vi "EEG Preprocessing.vi"() -> ()   [LabVIEW 2016]
uses:
  3. Features Extraction/_Feature Extraction Utility/_vlib/EF_FrequencyFilter.ctl
  3. Features Extraction/_Feature Extraction Utility/_vlib/EF_SpatialFilter.ctl
  _XML_EEG_File_Parser/_vlib/XML_EEG_File.lvclass
  <vilib>/xml/Load XML File.vi
  <vilib>/xml/NI_XML.lvlib
  3. Features Extraction/_Feature Extraction Utility/Feature Extraction.lvlib
panel:
  in  "Apply Settings":bool
  in  "Tab Control 2":T1(tab)=enum."Частотная фильтрация"
  in  "EOG channels":i32[](array[numeric])=[22, 23, 24] caption="Каналы с электроокулограммой (ЭОГ)" min=0 max=256 step=1
  in  "CSP params":path caption="Путь к файлу с параметрами CSP-фильтра"
  in  "SpatialFilter":T2=enum."Common Average Reference" caption="Метод пространственной фильтрации"
  in  "low cutoff freq":dbl=0.5 caption="Нижняя граница полосы пропускания, Гц"
  in  "high cutoff freq":dbl=50.0 caption="Верхняя граница полосы пропускания, Гц"
  in  "FrequencyFilter":T3 caption="Метод частотной фильтрации"
  in  "ReInit?":bool
  in  "Exit Button":bool
  in  "Tab Control":enum32{"Сигнал ЭЭГ", "Один канал"}(tab)
  out "Class Label":string caption="Метка класса"
  out "Dataset Number":i32 caption="Номер пробы"
  out "Raw EEG":dbl[][](graph) caption="Сигнал ЭЭГ (ориг.)"
  out "Preprocessed EEG":dbl[][](graph) caption="Сигнал ЭЭГ после предобработки"
  in  "Next Dataset":bool
  in  "Previous Dataset":bool
  out "Channel Name":string caption="Название канала"
  in  "Channel Number":i32 caption="Номер канала" min=0 max=24 step=1
  out "Wavelet Transform":dbl[][](graph) caption="Спектрограмма сигнала ЭЭГ (после предобработки)"
  out "Single Channel Preproc":dbl[](graph) caption="Сигнал ЭЭГ после предобработки"
  out "Single Channel Graph":dbl[](graph) caption="Сигнал ЭЭГ в одном канале"
  out "Spectrum":dbl[](graph) caption="Энергетический спектр сигнала ЭЭГ (после предобработки)"
  # "This VI is a part of BCI Design library, http://www.ru-bci.org \nCopyright © 2020, Sotnikov Peter, All rights reserved. License: GNU GPLv3"
  # "Предобработка"
  # "Параметры метода"
  # "Параметры метода"
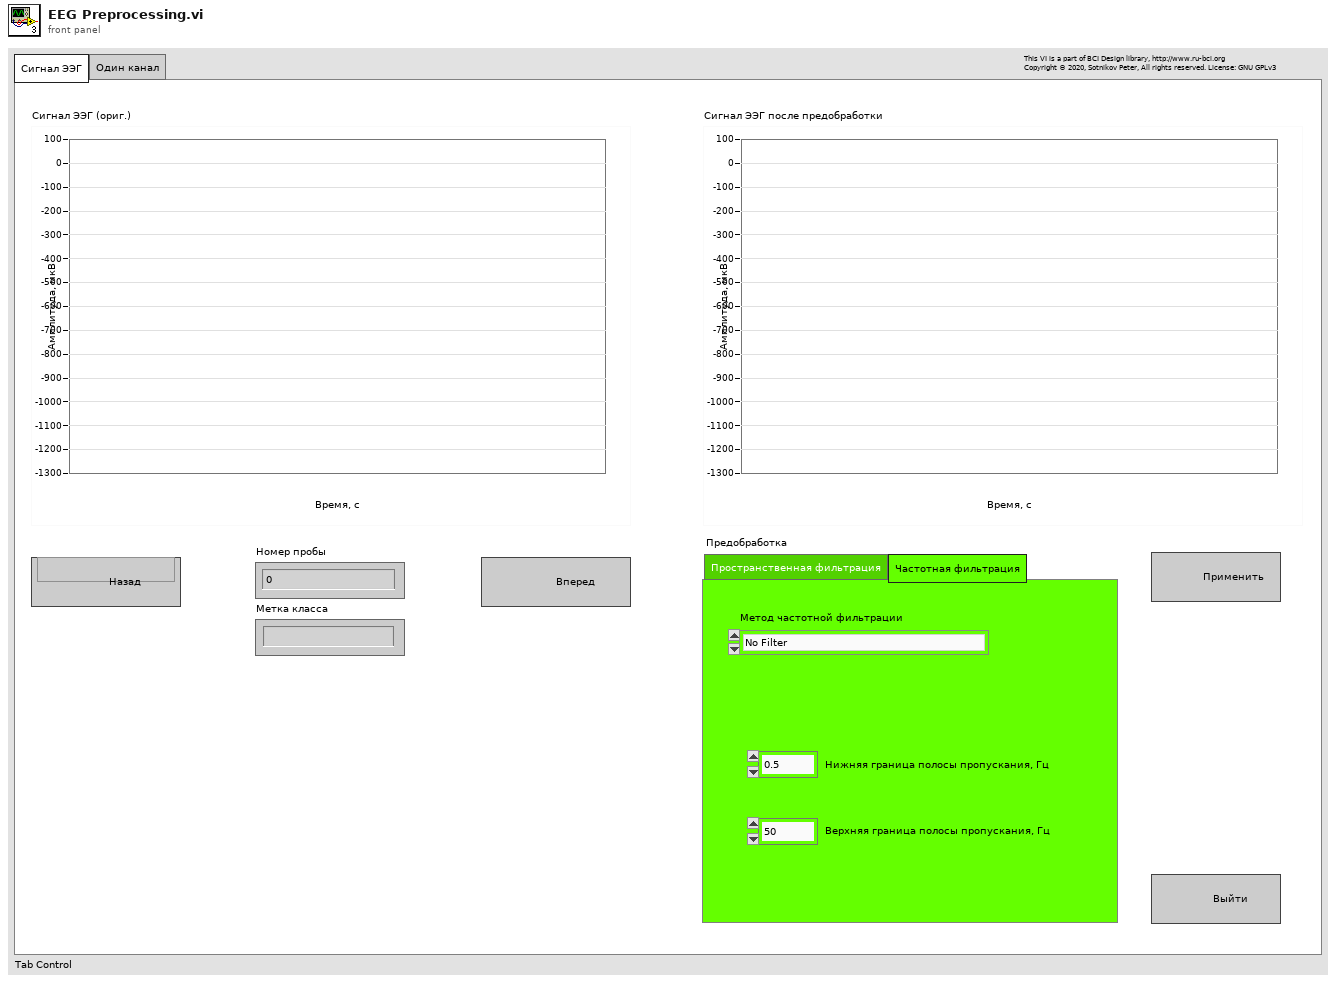
[diagram p1: front panel]
types:
  T1 = enum32{"Пространственная фильтрация", "Частотная фильтрация"}
  T2 = typedef "Feature Extraction.lvlib/EF_SpatialFilter.ctl" = enum16{"No Filter", "Common Average Reference", "Common Spatial Pattern Filter", "Removal of EOG Artifacts"}
  T3 = typedef "Feature Extraction.lvlib/EF_FrequencyFilter.ctl" = enum16{"No Filter", "Kaiser Filter"}
  T4 = typedef "XML_EEG_File_Parser.lvlib/XML_EEG_Header.ctl" = cluster{"Attributes":cluster{"ChannelDataType":string, "NumberOfChannels":i32, "SampleRateHz":dbl, "MarkerChannel":i32}, "Body":cluster{"PatientSpecificData":string, "NumberOfDatasets":i32, "Channels":string[]}}
  T5 = cluster{"SpatialFilter":T2, "CSP params":path, "FrequencyFilter":T3, "low cutoff freq":dbl, "high cutoff freq":dbl}
  T6 = typedef "XML_EEG_File_Parser.lvlib/XML_EEG_Dataset.ctl" = cluster{"Attributes":cluster{"NumberOfSamples":i32, "StartDateTime":timestamp}, "Body":cluster{"MarkerValue":string, "Channels":waveform(dbl)[]}}
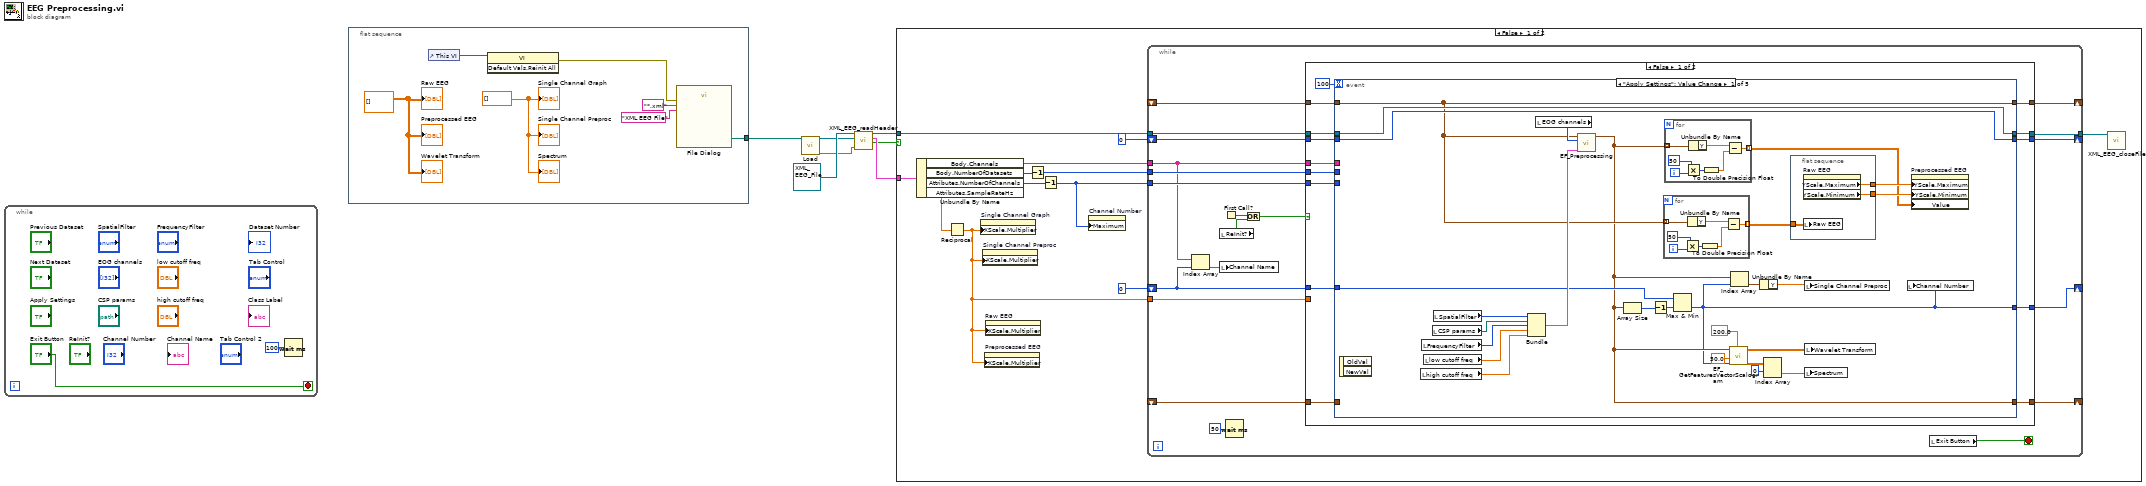
[diagram p0: block diagram]
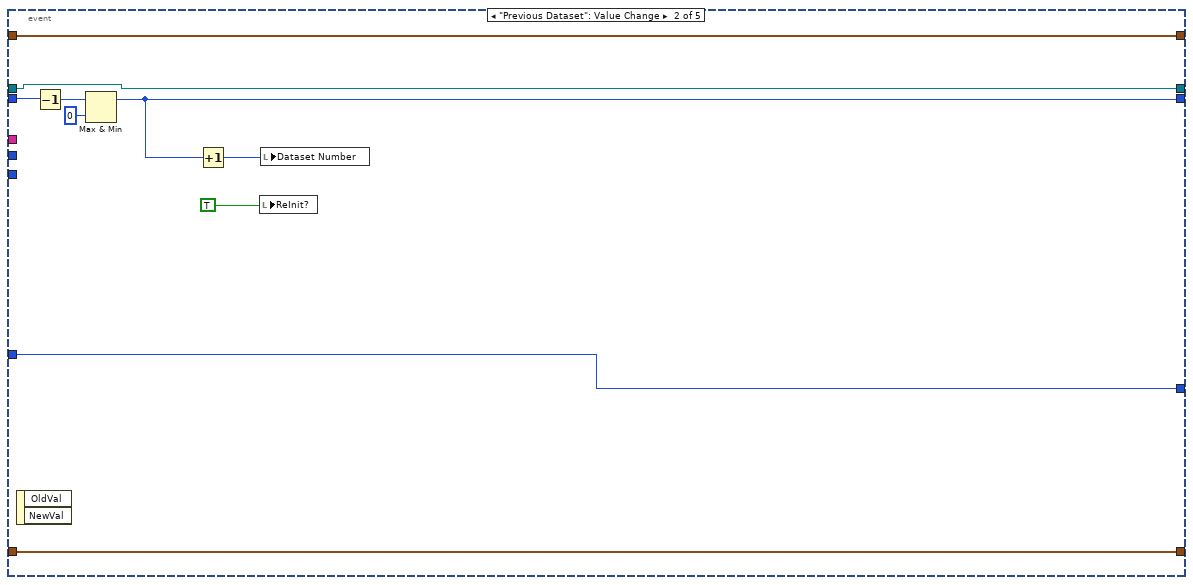
[diagram p2: hidden frame]
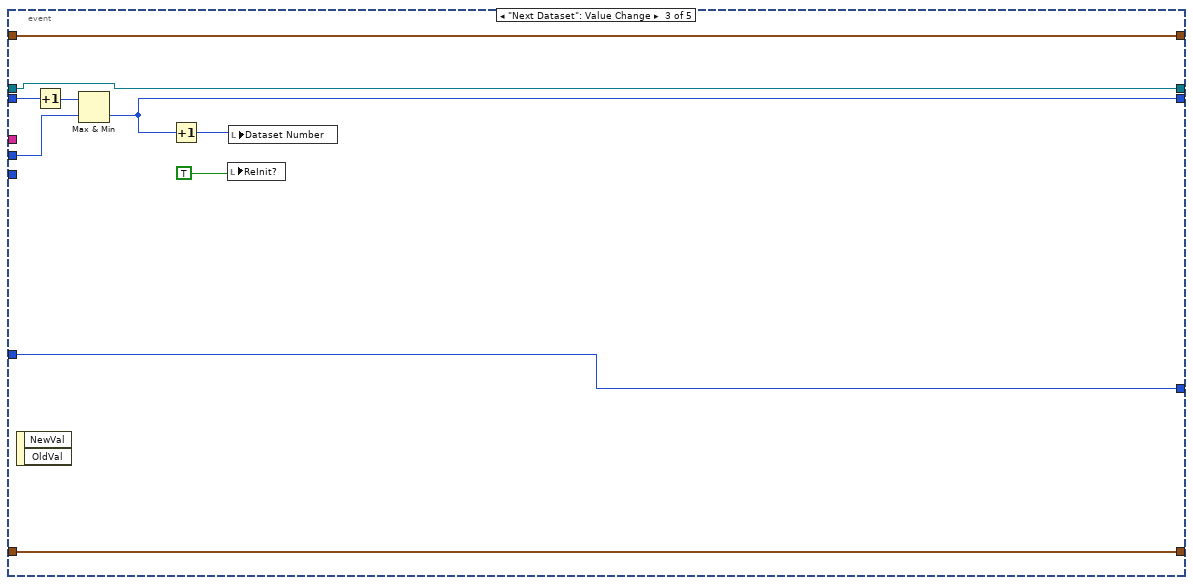
[diagram p3: hidden frame]
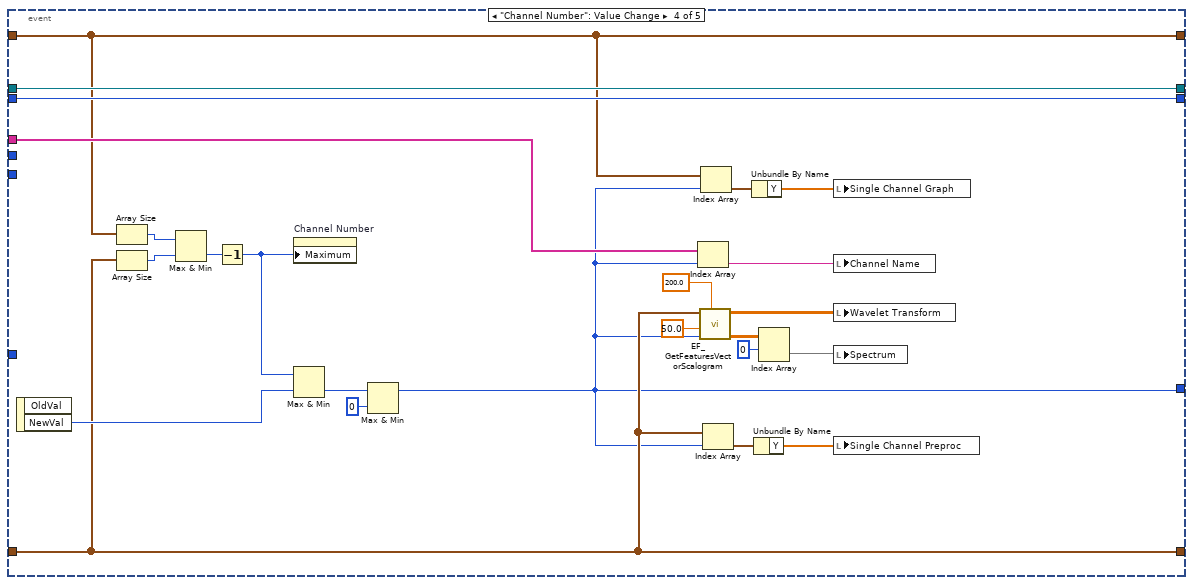
[diagram p4: hidden frame]
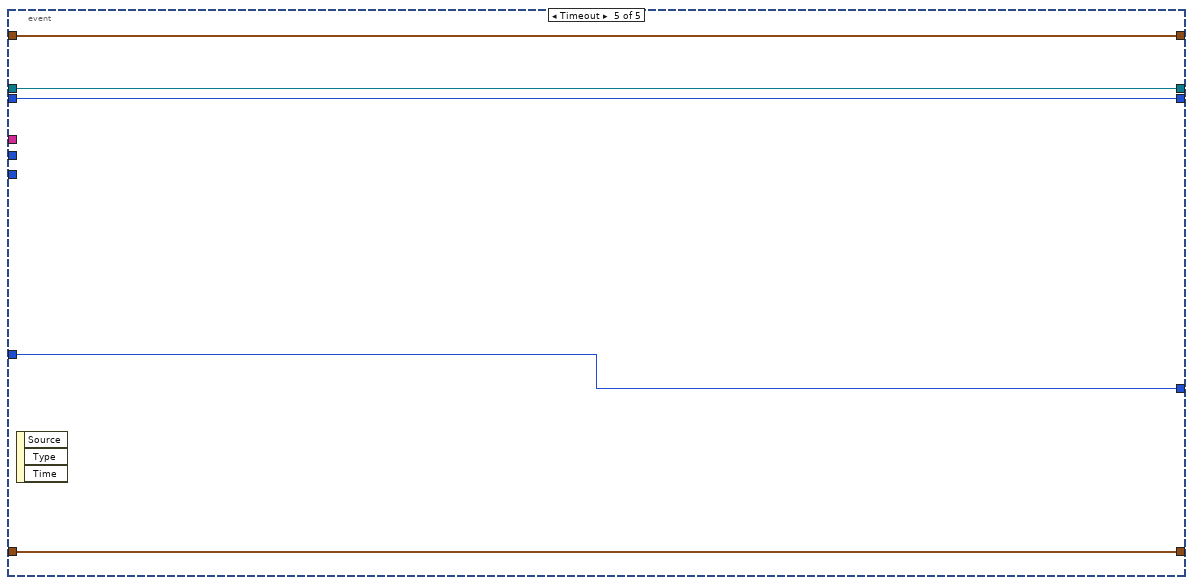
[diagram p5: hidden frame]
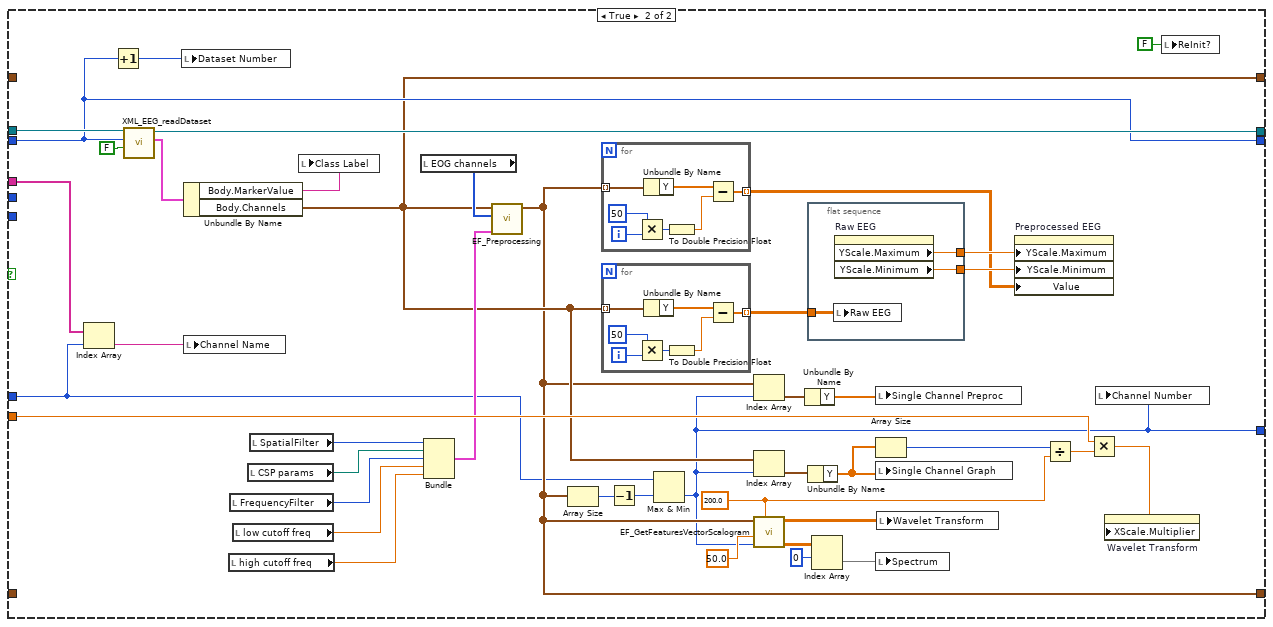
[diagram p6: hidden frame]
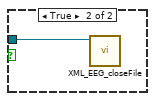
[diagram p7: hidden frame]
diagram:
  n1 = while {
    stop <- "Exit Button" stop-if-true
    n2 = Wait (ms)(milliseconds to wait=u32 100) -> ()  [unwired: 1 out]
  }
  n3 = flat-sequence {
    tunnel: [w11] -> w7
    frame #0 {
      w10 = dbl[] []
      w16 = dbl[][] []
      n4 = control-ref of="This VI"() -> (w13:refnum<vi>)
      n5 = invoke class="VI" method="Default Vals.Reinit All"(reference=w13) -> (error out=w12:errorcluster)  [unwired: 2 in, 2 out]
      n6 = call "File Dialog"("error in"=w12, "pattern (all files)"="*.xml", "pattern label"="XML EEG File") -> ("selected path"=w11:path)  [unwired: 9 in, 3 out]
      "Raw EEG" <- w16
      "Preprocessed EEG" <- w16
      "Single Channel Graph" <- w10
      "Single Channel Preproc" <- w10
      "Wavelet Transform" <- w16
      "Spectrum" <- w10
    }
  }
  n7 = call-poly <vilib>:"Load.vi"("path to XML document"=w7) -> ("DOM document out"=w5:refnum<k20>, "error out"=w4:errorcluster)  [unwired: 12 in, 1 out]
  n8 = call "XML_EEG_readHeader.vi"("error in (no error)"=w4, "DOM document in"=w5, "XML_EEG_Class in"=refnum<class "XML_EEG_File.lvclass"> refnum ("XML_EEG_File_Parser.lvlib:XML_EEG_File.lvclass")) -> ("Errors?"=w1:bool, "XML Header out"=w2:T4, "XML_EEG_Class out"=w3:refnum<class "XML_EEG_File.lvclass">)  [unwired: 6 in]
  n9 = case shown="False" w1 {
    tunnel: w3 -> [w28 w214]
    tunnel: w2 -> [w27 _]
    frame False {
      n10 = Unbundle By Name(w27) -> ("Body.Channels"=w20:string[], "Body.NumberOfDatasets"=w22:i32, "Attributes.NumberOfChannels"=w18:i32, "Attributes.SampleRateHz"=w23:dbl)
      n11 = Reciprocal(x=w23) -> (1/x=w19:dbl)
      n12 = property on="Single Channel Graph" class="WFGraph (strict)"("XScale.Multiplier"=w19) -> ()  [unwired: 2 in, 2 out]
      n13 = property on="Single Channel Preproc" class="WFGraph (strict)"("XScale.Multiplier"=w19) -> ()  [unwired: 2 in, 2 out]
      n14 = property on="Preprocessed EEG" class="WFGraph (strict)"("XScale.Multiplier"=w19) -> ()  [unwired: 2 in, 2 out]
      n15 = property on="Raw EEG" class="WFGraph (strict)"("XScale.Multiplier"=w19) -> ()  [unwired: 2 in, 2 out]
      n16 = Decrement(x=w22) -> (x-1=w21:i32)
      n17 = Decrement(x=w18) -> (x-1=w17:i32)
      n18 = property on="Channel Number" class="DigNum (strict)"("Maximum"=w17) -> ()  [unwired: 2 in, 2 out]
      n19 = while {
        tunnel: w28 -> [w48]
        shift-right: [w45] -> _
        shift-left: 0 -> [w47]
        tunnel: [w46] -> w25
        shift-right: [w42] -> _
        shift-left: 0 -> [w31]
        shift-right: [w41] -> _
        shift-left: _ -> [w40]
        shift-right: [w39] -> _
        shift-left: _ -> [w38]
        tunnel: w21 -> [w37]
        tunnel: w17 -> [w36]
        tunnel: w20 -> [w30]
        tunnel: w19 -> [w35]
        stop <- w44 stop-if-true
        n20 = Index Array(array=w30, index=w31) -> (element=w29:string)
        n21 = local read "ReInit?"() -> (w33:bool)
        n22 = local write "Channel Name"(w29) -> ()
        n23 = First Call?() -> (First Call?: T/F=w34:bool)
        n24 = Wait (ms)(milliseconds to wait=u32 50) -> ()  [unwired: 1 out]
        n25 = Or(x=w34, y=w33) -> (x .or. y?=w32:bool)
        n26 = case shown="False" w32 {
          tunnel: w48 -> [w54 w196]
          tunnel: w47 -> [w55 w190]
          tunnel: [w53 w194] -> w46
          tunnel: [w56 w190] -> w45
          tunnel: w31 -> [w58 w157]
          tunnel: [w57 w156] -> w42
          tunnel: [w59 w165] -> w41
          tunnel: w40 -> [w60 _]
          tunnel: [w61 w158] -> w39
          tunnel: w38 -> [w62 _]
          tunnel: w37 -> [w51 _]
          tunnel: w36 -> [w50 _]
          tunnel: w30 -> [w49 w177]
          tunnel: w35 -> [_ w171]
          frame False {
            n27 = event shown="[0] \"Apply Settings\": Value Change" {
              selector: _ -> [_ _ _ _ _]
              dyn-events: _ -> [_ _ _ _ _]
              timeout: 100 -> [_ _ _ _ _]
              tunnel: w62 -> [_ w113 w125 w132 w151]
              tunnel: [w66 w113 w125 w132 w151] -> w61
              tunnel: w60 -> [w72 w109 w119 w133 w155]
              tunnel: [w72 w109 w119 w133 w155] -> w59
              tunnel: w58 -> [w67 w112 w123 _ w152]
              tunnel: [w63 w112 w123 w127 w152] -> w57
              tunnel: [w76 w111 w120 w142 w153] -> w56
              tunnel: w55 -> [w76 w116 w126 w142 w153]
              tunnel: w54 -> [w75 w107 w118 w141 w154]
              tunnel: [w75 w107 w118 w141 w154] -> w53
              tunnel: w51 -> [_ _ w122 _ _]
              tunnel: w50 -> [_ _ _ _ _]
              tunnel: w49 -> [_ _ _ w136 _]
              event "Apply Settings": Value Change {
                n28 = event-data() -> ()  [unwired: 1 in, 2 out]
                n29 = local read "high cutoff freq"() -> (w80:dbl)
                n30 = local read "FrequencyFilter"() -> (w82:T3)
                n31 = local read "low cutoff freq"() -> (w81:dbl)
                n32 = local read "CSP params"() -> (w83:path)
                n33 = local read "SpatialFilter"() -> (w84:T2)
                n34 = Bundle("SpatialFilter"=w84, "CSP params"=w83, "FrequencyFilter"=w82, "low cutoff freq"=w81, "high cutoff freq"=w80) -> (w89:T5)  [unwired: 1 in]
                n35 = local read "EOG channels"() -> (w73:i32[])
                n36 = call "EF_Preprocessing.vi"("Preprocessing params"=w89, "EOG channels"=w73, "EEG data in"=w72) -> ("EEG data out"=w66:waveform(dbl)[])  [unwired: 8 in]
                n37 = Array Size(array=w66) -> (size(s)=w65:i32)
                n38 = Decrement(x=w65) -> (x-1=w64:i32)
                n39 = for {
                  tunnel: w72 -> [w99] mode=indexing
                  tunnel: [w93] -> w71 mode=indexing
                  i -> [w98]
                  n40 = Multiply(x=50, y=w98) -> (x*y=w95:i32)
                  n41 = Unbundle By Name(w99) -> ("Y"=w96:dbl[])
                  n42 = To Double Precision Float(number=w95) -> (double precision float=w94:dbl)
                  n43 = Subtract(x=w96, y=w94) -> (x-y=w93:dbl[])
                }
                n44 = for {
                  tunnel: w66 -> [w106] mode=indexing
                  tunnel: [w100] -> w68 mode=indexing
                  i -> [w105]
                  n45 = Multiply(x=50, y=w105) -> (x*y=w102:i32)
                  n46 = Unbundle By Name(w106) -> ("Y"=w103:dbl[])
                  n47 = To Double Precision Float(number=w102) -> (double precision float=w101:dbl)
                  n48 = Subtract(x=w103, y=w101) -> (x-y=w100:dbl[])
                }
                n49 = Max & Min(x=w67, y=w64) -> (min(x,y)=w63:i32)  [unwired: 1 out]
                n50 = call "EF_GetFeaturesVectorScalogram.vi"("TimeShiftsNum"=200.0, "ChannelNumber"=w63, "High cutoff frequency"=50.0 ("TimeShiftsNum"), "Array Of Waveforms in"=w66) -> ("StackedSpectra"=w86:dbl[][], "StackedScalograms"=w78:dbl[][])  [unwired: 5 in, 1 out]
                n51 = Index Array(array=w66, index=w63) -> (element=w88:waveform(dbl))
                n52 = Unbundle By Name(w88) -> ("Y"=w79:dbl[])
                n53 = Index Array(array=w86, index (row)=0) -> (element=w77:dbl[])  [unwired: 1 in]
                n54 = flat-sequence {
                  tunnel: w71 -> [w92]
                  tunnel: [w91] -> w70
                  tunnel: [w90] -> w69
                  frame #0 {
                    n55 = property on="Raw EEG" class="WFGraph (strict)"() -> ("YScale.Maximum"=w90:dbl, "YScale.Minimum"=w91:dbl)  [unwired: 2 in, 2 out]
                    n56 = local write "Raw EEG"(w92) -> ()
                  }
                }
                n57 = local write "Single Channel Preproc"(w79) -> ()
                n58 = local write "Spectrum"(w77) -> ()
                n59 = local write "Wavelet Transform"(w78) -> ()
                n60 = local write "Channel Number"(w63) -> ()
                n61 = property on="Preprocessed EEG" class="WFGraph (strict)"("YScale.Maximum"=w69, "YScale.Minimum"=w70, "Value"=w68) -> ()  [unwired: 2 in, 2 out]
              }
              event "Previous Dataset": Value Change {
                n62 = event-data() -> ()  [unwired: 1 in, 2 out]
                n63 = Decrement(x=w116) -> (x-1=w115:i32)
                n64 = Max & Min(x=w115, y=0) -> (max(x,y)=w111:i32)  [unwired: 1 out]
                n65 = Increment(x=w111) -> (x+1=w110:i32)
                n66 = local write "ReInit?"(TRUE ("Add offset?")) -> ()
                n67 = local write "Dataset Number"(w110) -> ()
              }
              event "Next Dataset": Value Change {
                n68 = event-data() -> ()  [unwired: 1 in, 2 out]
                n69 = Increment(x=w126) -> (x+1=w121:i32)
                n70 = Max & Min(x=w121, y=w122) -> (min(x,y)=w120:i32)  [unwired: 1 out]
                n71 = Increment(x=w120) -> (x+1=w124:i32)
                n72 = local write "ReInit?"(TRUE ("Add offset?")) -> ()
                n73 = local write "Dataset Number"(w124) -> ()
              }
              event "Channel Number": Value Change {
                n74 = event-data() -> ("NewVal"=w150:i32)  [unwired: 1 in, 1 out]
                n75 = Array Size(array=w133) -> (size(s)=w130:i32)
                n76 = Array Size(array=w132) -> (size(s)=w131:i32)
                n77 = Max & Min(x=w130, y=w131) -> (min(x,y)=w129:i32)  [unwired: 1 out]
                n78 = Decrement(x=w129) -> (x-1=w128:i32)
                n79 = property on="Channel Number" class="DigNum (strict)"("Maximum"=w128) -> ()  [unwired: 2 in, 2 out]
                n80 = Max & Min(x=w128, y=w150) -> (min(x,y)=w149:i32)  [unwired: 1 out]
                n81 = Max & Min(x=w149, y=0) -> (max(x,y)=w127:i32)  [unwired: 1 out]
                n82 = Index Array(array=w136, index=w127) -> (element=w135:string)
                n83 = call "EF_GetFeaturesVectorScalogram.vi"("TimeShiftsNum"=200.0, "ChannelNumber"=w127, "High cutoff frequency"=50.0 ("TimeShiftsNum"), "Array Of Waveforms in"=w132) -> ("StackedSpectra"=w145:dbl[][], "StackedScalograms"=w139:dbl[][])  [unwired: 5 in, 1 out]
                n84 = Index Array(array=w133, index=w127) -> (element=w147:waveform(dbl))
                n85 = Index Array(array=w132, index=w127) -> (element=w143:waveform(dbl))
                n86 = Unbundle By Name(w147) -> ("Y"=w140:dbl[])
                n87 = Unbundle By Name(w143) -> ("Y"=w137:dbl[])
                n88 = Index Array(array=w145, index (row)=0) -> (element=w138:dbl[])  [unwired: 1 in]
                n89 = local write "Single Channel Graph"(w140) -> ()
                n90 = local write "Channel Name"(w135) -> ()
                n91 = local write "Wavelet Transform"(w139) -> ()
                n92 = local write "Spectrum"(w138) -> ()
                n93 = local write "Single Channel Preproc"(w137) -> ()
              }
              event Timeout {
                n94 = event-data() -> ()  [unwired: 1 in, 3 out]
              }
            }
          }
          frame True {
            w169 = 200.0 ("TimeShiftsNum")
            n95 = Index Array(array=w177, index=w157) -> (element=w176:string)
            n96 = Increment(x=w190) -> (x+1=w195:i32)
            n97 = call "XML_EEG_readDataset.vi"("Add offset?"=FALSE, "DatasetNumber"=w190, "XML_EEG_File in"=w196) -> ("XML Dataset out"=w193:T6, "XML_EEG_File out"=w194:refnum<class "XML_EEG_File.lvclass">)  [unwired: 6 in, 1 out]
            n98 = local write "Dataset Number"(w195) -> ()
            n99 = Unbundle By Name(w193) -> ("Body.MarkerValue"=w192:string, "Body.Channels"=w165:waveform(dbl)[])
            n100 = local write "Channel Name"(w176) -> ()
            n101 = local read "high cutoff freq"() -> (w185:dbl)
            n102 = local read "FrequencyFilter"() -> (w187:T3)
            n103 = local read "low cutoff freq"() -> (w186:dbl)
            n104 = local read "CSP params"() -> (w188:path)
            n105 = local read "SpatialFilter"() -> (w189:T2)
            n106 = local write "Class Label"(w192) -> ()
            n107 = local read "EOG channels"() -> (w167:i32[])
            n108 = Bundle("SpatialFilter"=w189, "CSP params"=w188, "FrequencyFilter"=w187, "low cutoff freq"=w186, "high cutoff freq"=w185) -> (w166:T5)  [unwired: 1 in]
            n109 = call "EF_Preprocessing.vi"("Preprocessing params"=w166, "EOG channels"=w167, "EEG data in"=w165) -> ("EEG data out"=w158:waveform(dbl)[])  [unwired: 8 in]
            n110 = Array Size(array=w158) -> (size(s)=w160:i32)
            n111 = for {
              tunnel: w158 -> [w213] mode=indexing
              tunnel: [w207] -> w161 mode=indexing
              i -> [w212]
              n112 = Multiply(x=50, y=w212) -> (x*y=w209:i32)
              n113 = Unbundle By Name(w213) -> ("Y"=w210:dbl[])
              n114 = To Double Precision Float(number=w209) -> (double precision float=w208:dbl)
              n115 = Subtract(x=w210, y=w208) -> (x-y=w207:dbl[])
            }
            n116 = for {
              tunnel: w165 -> [w206] mode=indexing
              tunnel: [w200] -> w164 mode=indexing
              i -> [w205]
              n117 = Multiply(x=50, y=w205) -> (x*y=w202:i32)
              n118 = Unbundle By Name(w206) -> ("Y"=w203:dbl[])
              n119 = To Double Precision Float(number=w202) -> (double precision float=w201:dbl)
              n120 = Subtract(x=w203, y=w201) -> (x-y=w200:dbl[])
            }
            n121 = Decrement(x=w160) -> (x-1=w159:i32)
            n122 = Max & Min(x=w157, y=w159) -> (min(x,y)=w156:i32)  [unwired: 1 out]
            n123 = Index Array(array=w158, index=w156) -> (element=w184:waveform(dbl))
            n124 = Index Array(array=w165, index=w156) -> (element=w182:waveform(dbl))
            n125 = call "EF_GetFeaturesVectorScalogram.vi"("TimeShiftsNum"=w169, "ChannelNumber"=w156, "High cutoff frequency"=50.0, "Array Of Waveforms in"=w158) -> ("StackedSpectra"=w181:dbl[][], "StackedScalograms"=w178:dbl[][])  [unwired: 5 in, 1 out]
            n126 = Unbundle By Name(w184) -> ("Y"=w183:dbl[])
            n127 = flat-sequence {
              tunnel: w164 -> [w199]
              tunnel: [w198] -> w163
              tunnel: [w197] -> w162
              frame #0 {
                n128 = local write "Raw EEG"(w199) -> ()
                n129 = property on="Raw EEG" class="WFGraph (strict)"() -> ("YScale.Maximum"=w198:dbl, "YScale.Minimum"=w197:dbl)  [unwired: 2 in, 2 out]
              }
            }
            n130 = Unbundle By Name(w182) -> ("Y"=w175:dbl[])
            n131 = Index Array(array=w181, index (row)=0) -> (element=w179:dbl[])  [unwired: 1 in]
            n132 = local write "Single Channel Preproc"(w183) -> ()
            n133 = Array Size(array=w175) -> (size(s)=w174:i32)
            n134 = local write "Single Channel Graph"(w175) -> ()
            n135 = local write "Spectrum"(w179) -> ()
            n136 = local write "Wavelet Transform"(w178) -> ()
            n137 = property on="Preprocessed EEG" class="WFGraph (strict)"("YScale.Maximum"=w163, "YScale.Minimum"=w162, "Value"=w161) -> ()  [unwired: 2 in, 2 out]
            n138 = Divide(x=w174, y=w169) -> (x/y=w172:dbl)
            n139 = Multiply(x=w171, y=w172) -> (x*y=w173:dbl)
            n140 = local write "Channel Number"(w156) -> ()
            n141 = property on="Wavelet Transform" class="IntGraph (strict)"("XScale.Multiplier"=w173) -> ()  [unwired: 2 in, 2 out]
            n142 = local write "ReInit?"(FALSE ("ReInit?")) -> ()
          }
        }
        n143 = local read "Exit Button"() -> (w44:bool)
      }
      n144 = call "XML_EEG_closeFile.vi"("XML_EEG_File.lvclass"=w25) -> ()  [unwired: 10 in, 1 out]
    }
    frame True {
      n145 = call "XML_EEG_closeFile.vi"("XML_EEG_File.lvclass"=w214) -> ()  [unwired: 10 in, 1 out]
    }
  }
